vi "UI.vi"(0 "reference in":refnum<class "GUI Script Player.lvclass">, 5 "error in (no error)":errorcluster) -> (14 "reference out":refnum<class "GUI Script Player.lvclass">, 19 "error out":errorcluster)   [LabVIEW 2019, in "GUI Script Player.lvclass"]
uses:
  GUI Script Player.lvclass
  C:/Users/H4001/Documents/GitHub/H4000/src/GUI_class/GUI.lvclass
  GUI_class/GUI.lvclass/GUI.ctl
  ConfigJSON_class/ConfigJSON.lvclass
  TypeDef/Script.ctl
  TypeDef/Step.ctl
  TypeDef/Direction.ctl
  ConfigJSON_class/ConfigJSON.lvclass/ConfigJSON.ctl
  e526d8fc-7282-4644-9dda-8724ecf4fc0a.vi
  GUI_class/Set Win State.vi
  GUI_class/protected/GetSheredData.vi
  GUI_class/GUI.lvclass
panel:
  in  "Stop Button":bool
  in  "Start Button":bool
  out "String Indicator 2":string="Шаг 12/125"
  out "Horizontal Fill Indicator":dbl(slide)=29.646017699115045 scale=0.0..100.0
  out "XY Graph - Dark":cluster{"X":dbl[], "Y":dbl[]}[](graph) caption="Давление"
  out "Program name":string="Название"
  in  "Open":bool
  out "Steps":i32(listbox)
  # "Воспроизведение сценариев"
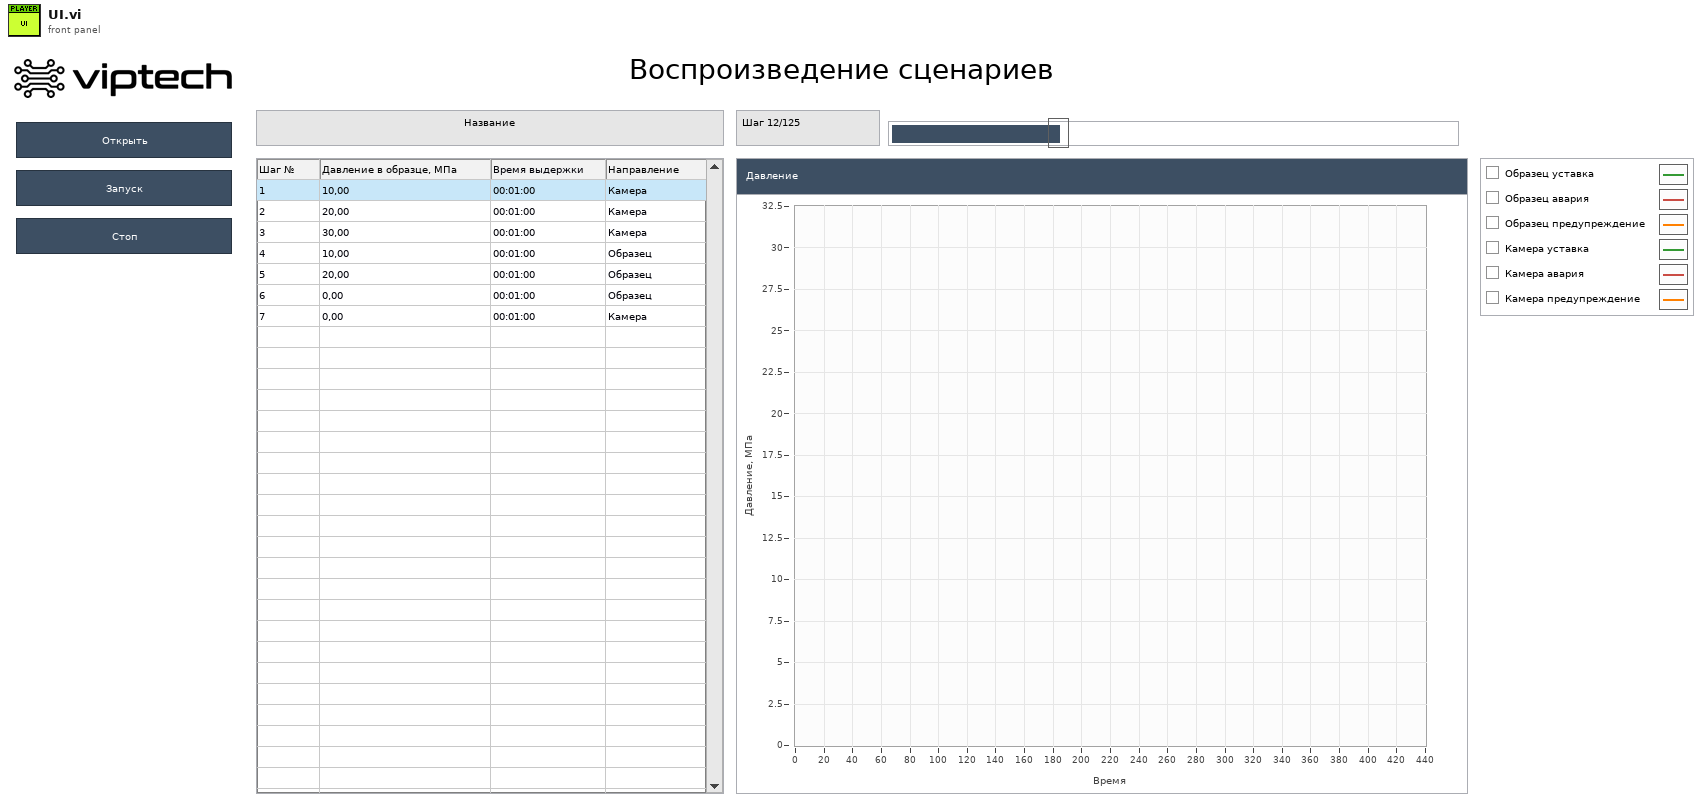
[diagram p1: front panel]
types:
  T1 = typedef "Script.ctl" = cluster{"Steps":T2[]}
  T2 = typedef "Step.ctl" = cluster{"Direction":T3, "Pressure MPa":dbl, "Time s":dbl, "Delta alarm MPa":dbl, "Delta warning MPa":dbl}
  T3 = typedef "Direction.ctl" = enum16{"None", "Chamber", "DUT"}
  T4 = enum32{"Invalid", "Standard", "Closed", "Hidden", "Minimized", "Maximized"}
  T5 = enum32{"invalid app kind", "Development System", "Run Time System", "Student Edition", "Embedded LabVIEW", "Evaluation", "Custom"}
  T6 = cluster{"Core":cluster{"Current VI Reference":refnum<vi>, "Close Panel on Exit?":bool}, "Dir Scripts":path, "Curr Script":T1, "selected path":path, "Steps ref":refnum<vi>}
  T7 = cluster{"Current VI Reference":refnum<vi>, "Close Panel on Exit?":bool}
  T8 = typedef "GUI Paths.ctl" = cluster{"Dir Data":path, "Dir Setting":path, "SensorLib":path, "Dir Scripts":path}
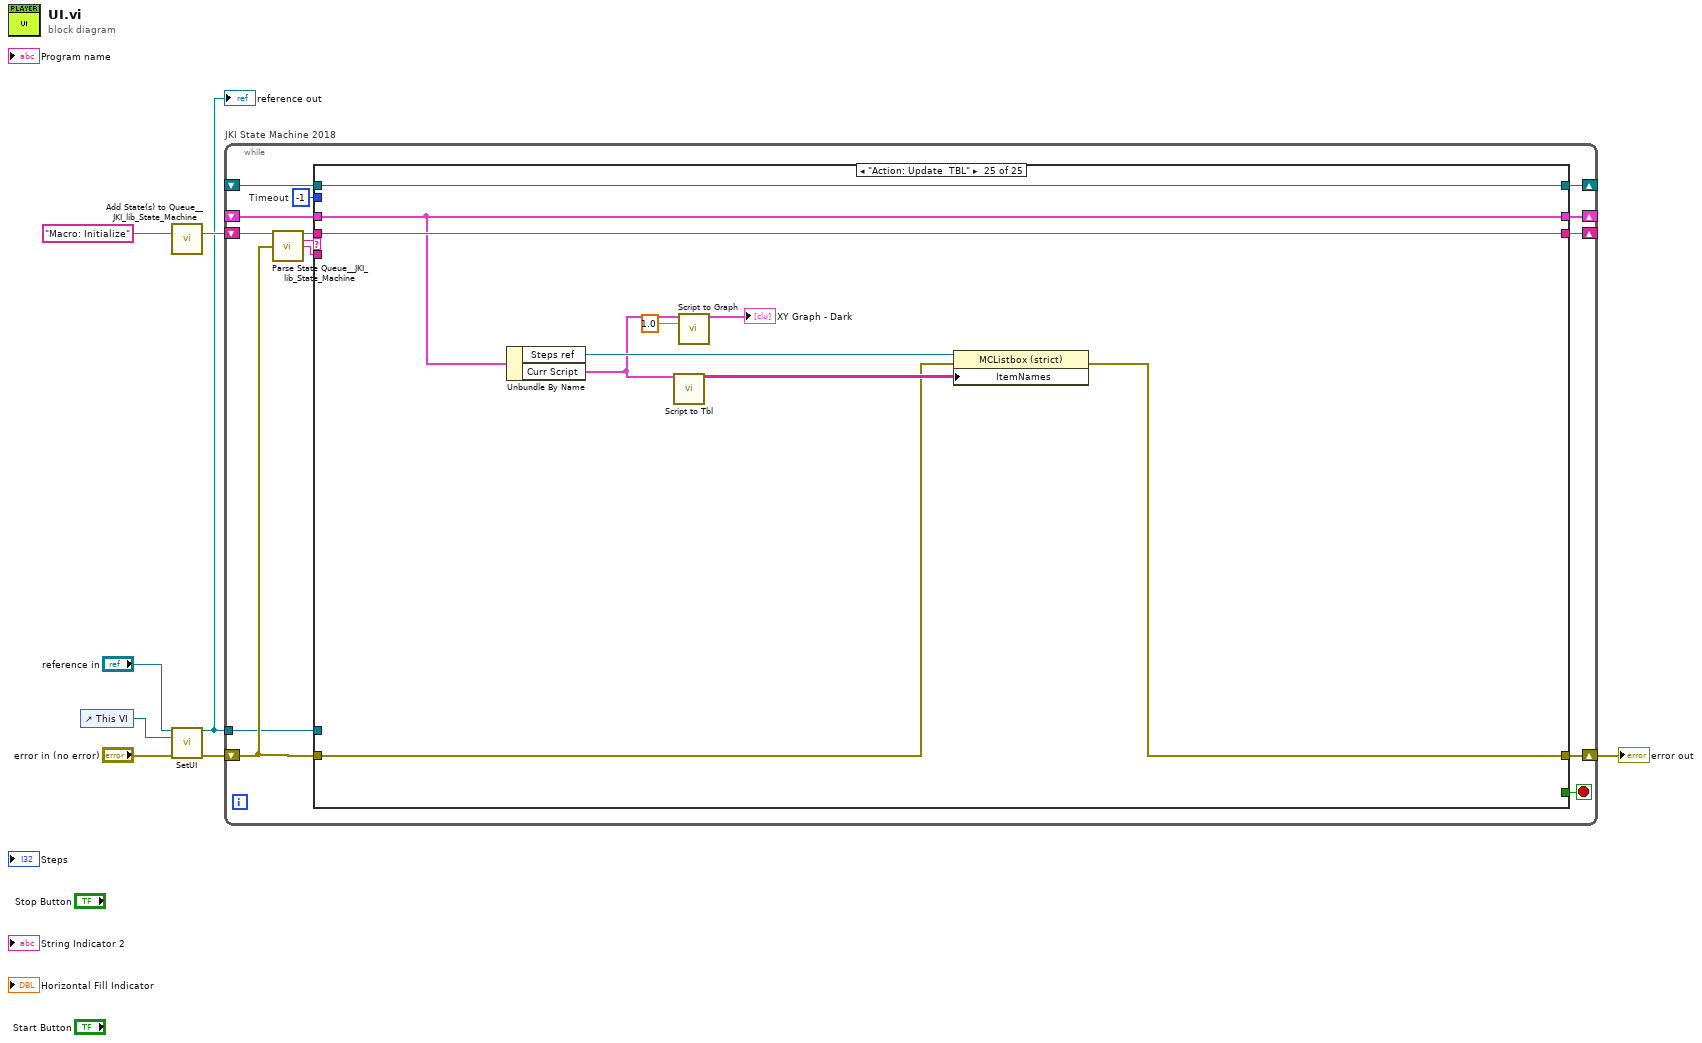
[diagram p0: block diagram]
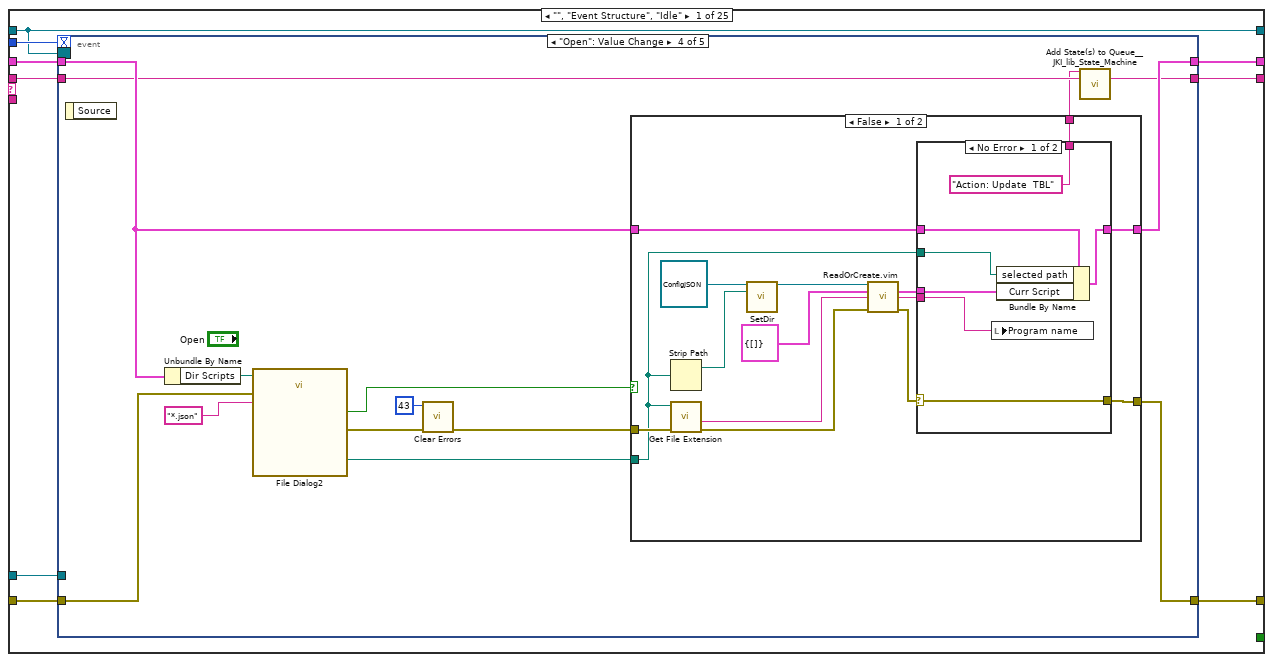
[diagram p2: hidden frame]
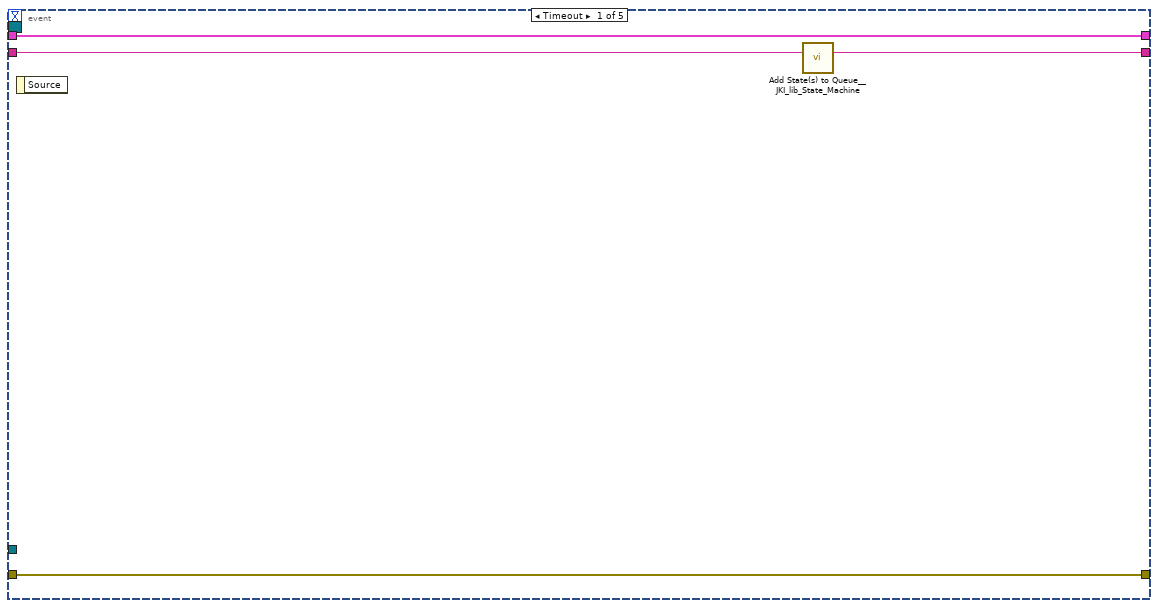
[diagram p3: hidden frame]
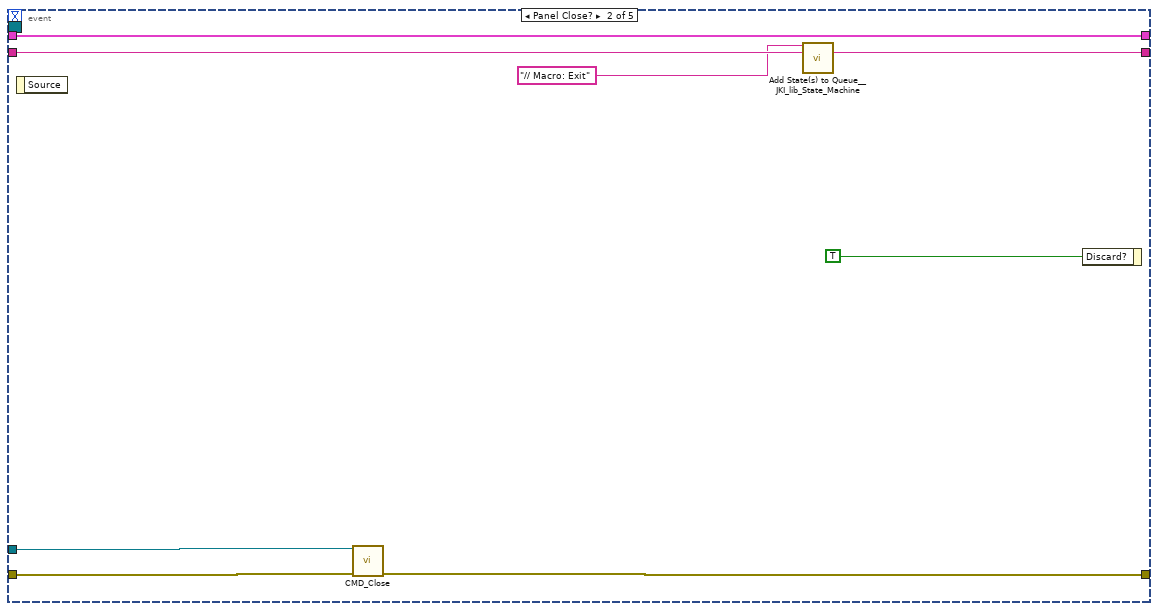
[diagram p4: hidden frame]
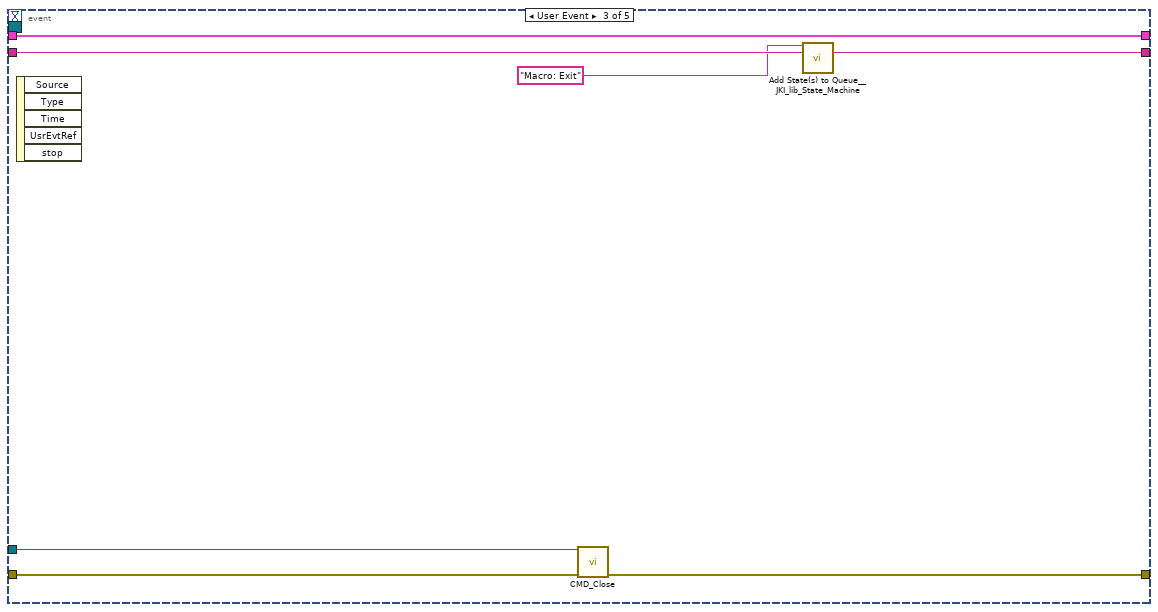
[diagram p5: hidden frame]
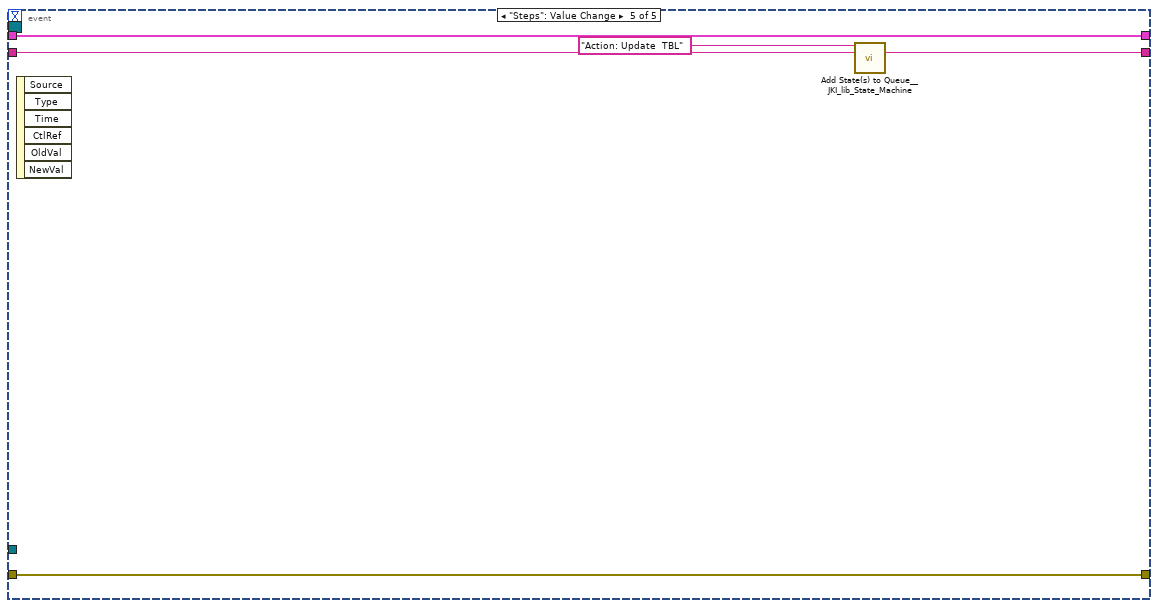
[diagram p8: hidden frame]
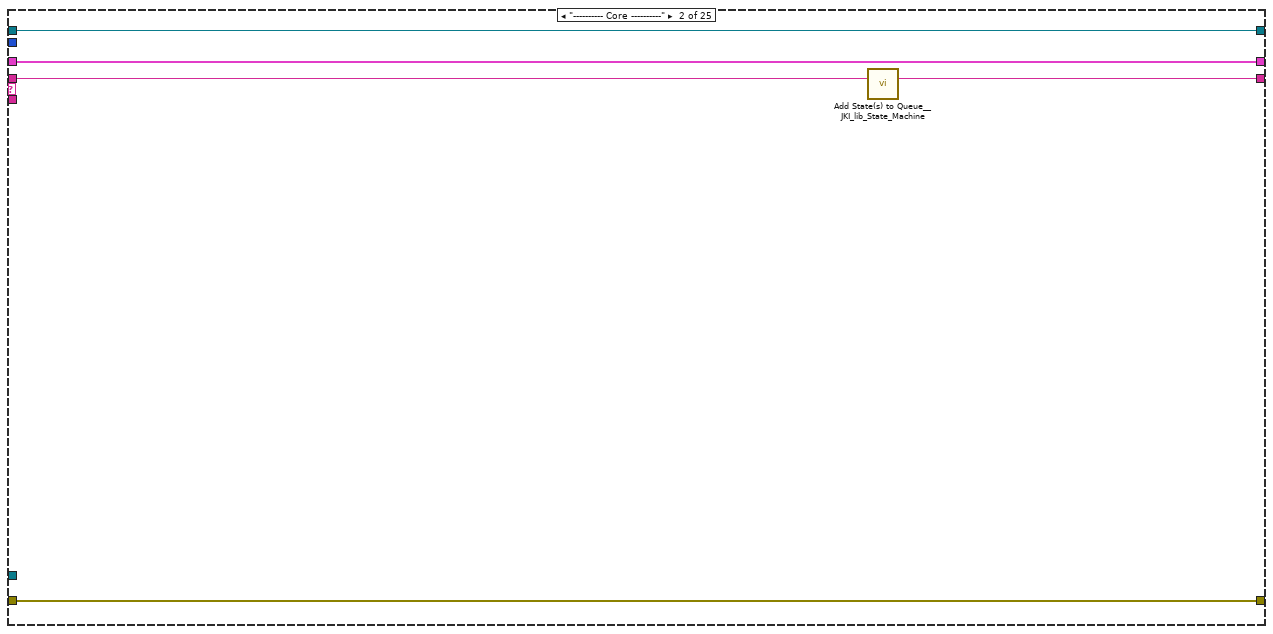
[diagram p9: hidden frame]
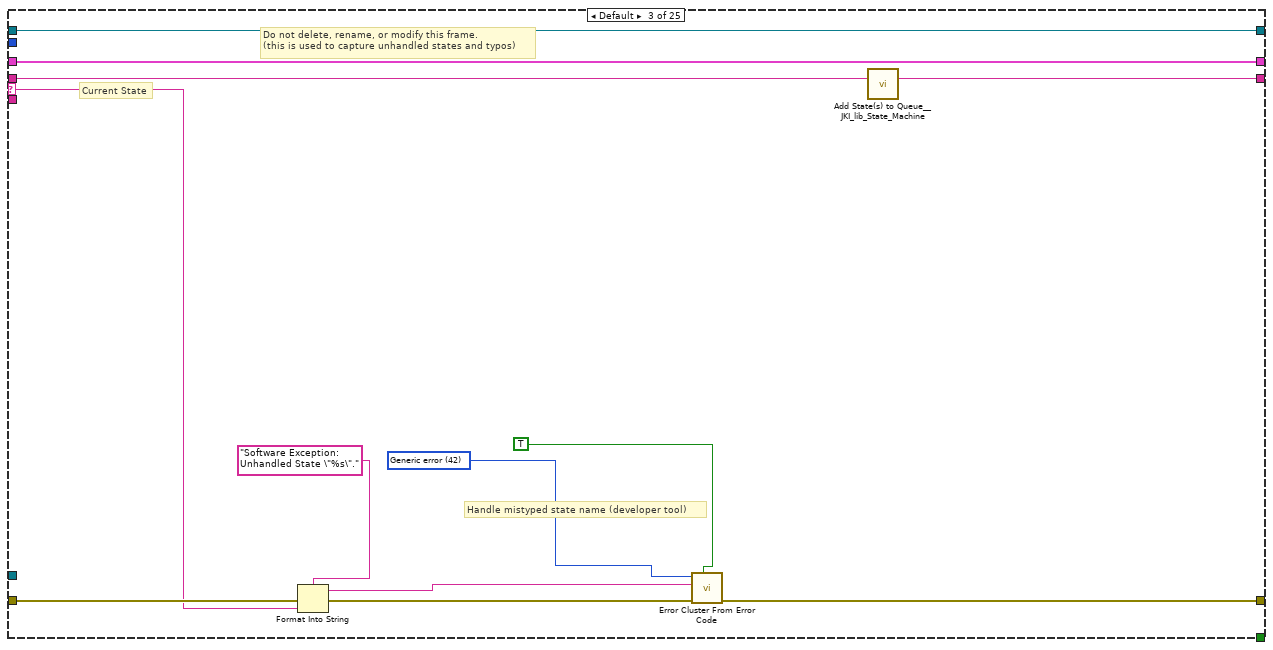
[diagram p10: hidden frame]
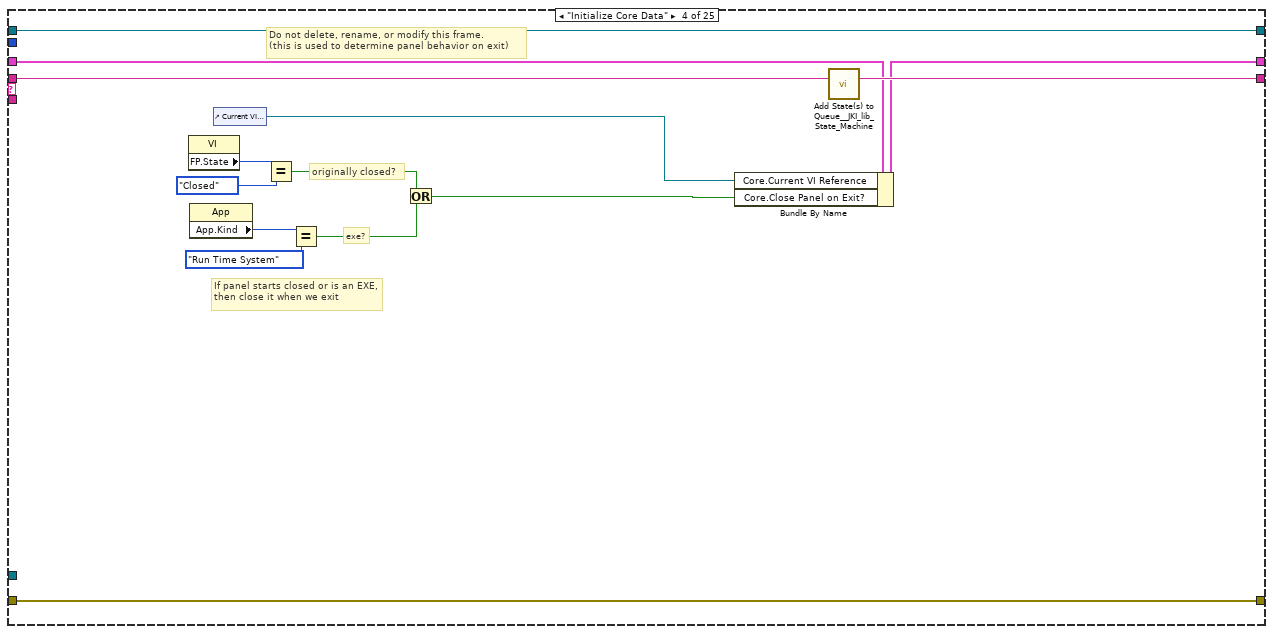
[diagram p11: hidden frame]
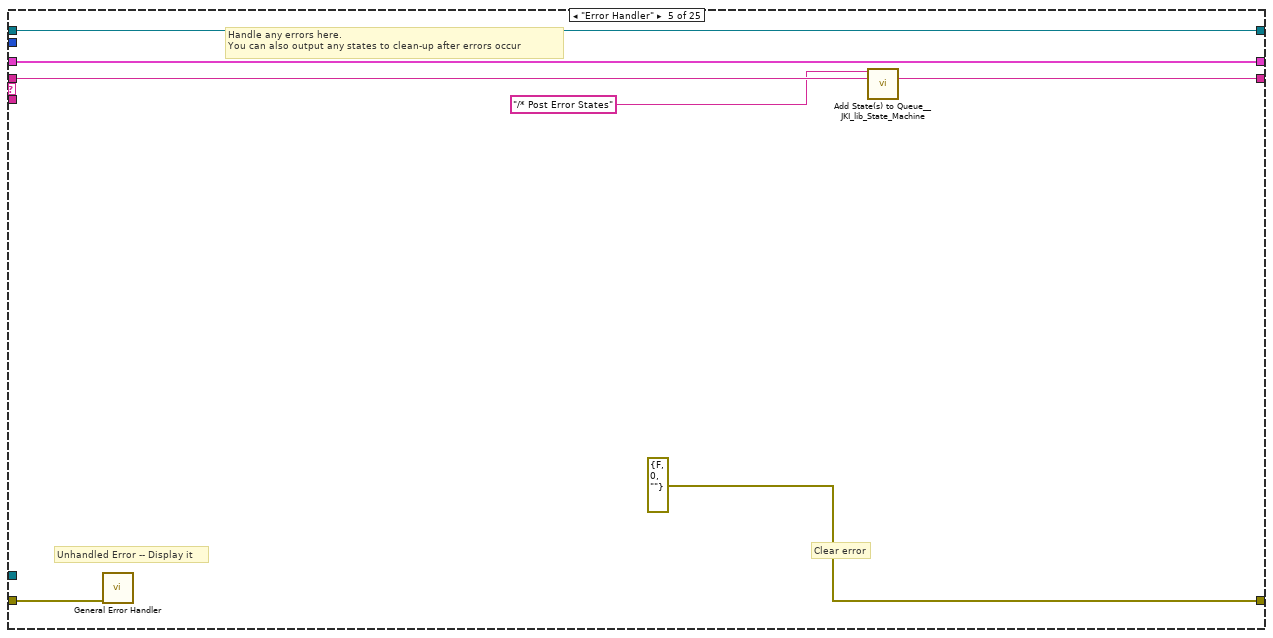
[diagram p12: hidden frame]
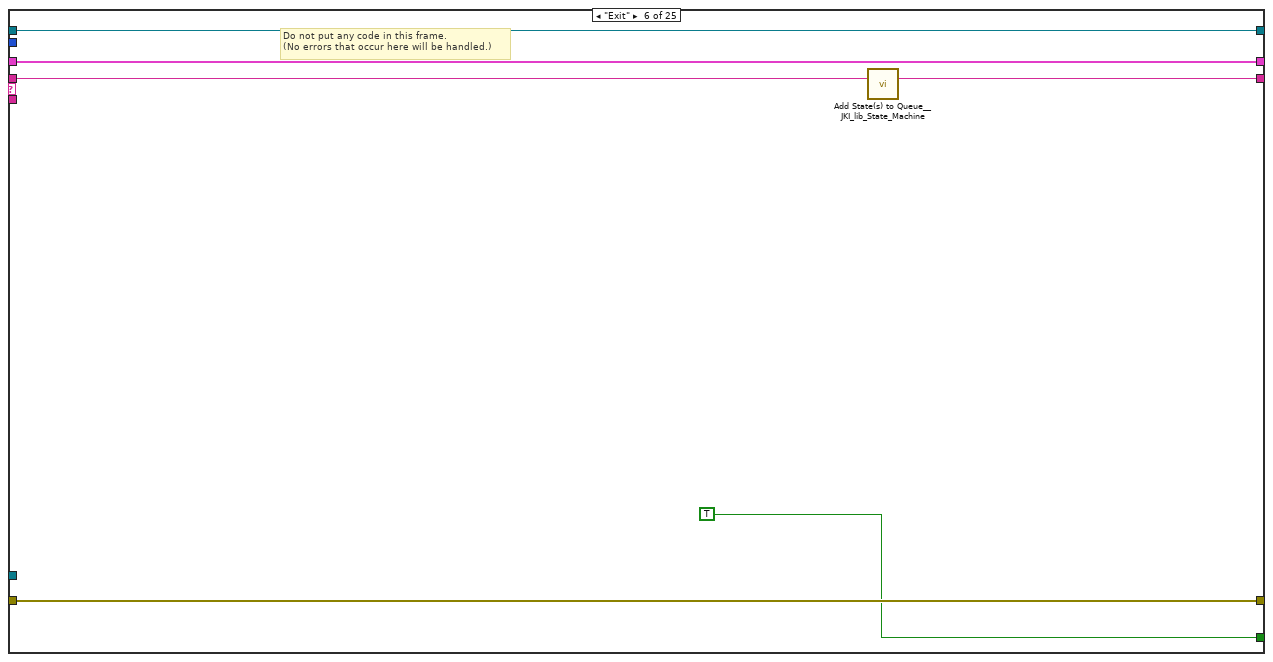
[diagram p13: hidden frame]
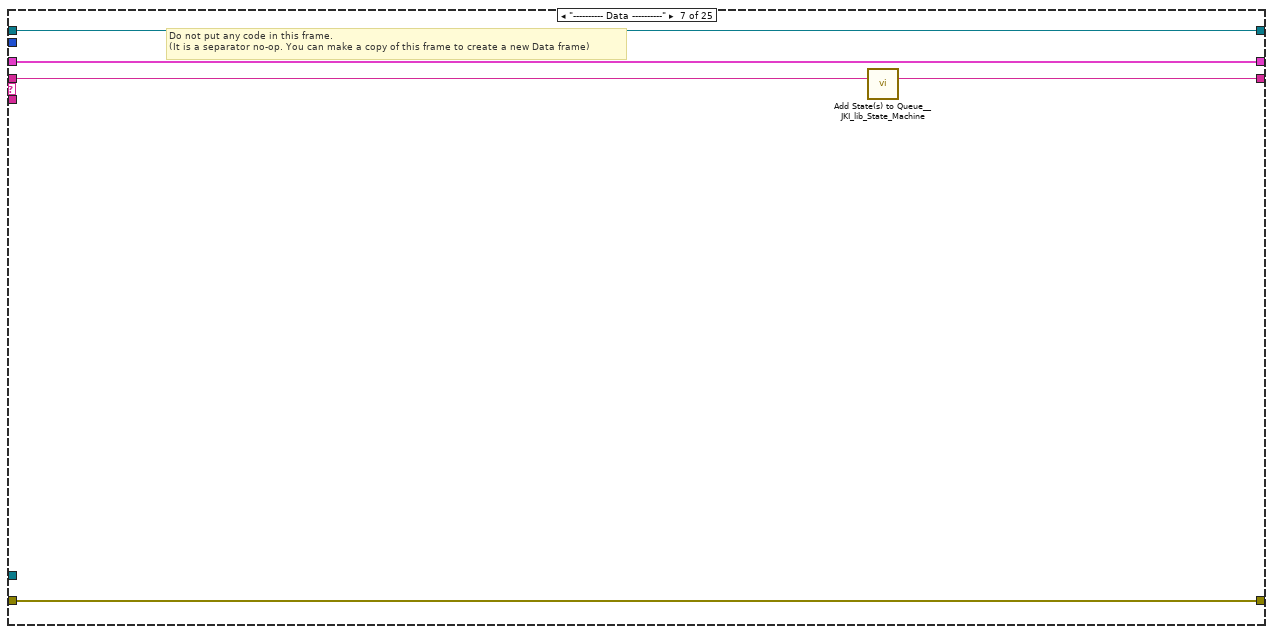
[diagram p14: hidden frame]
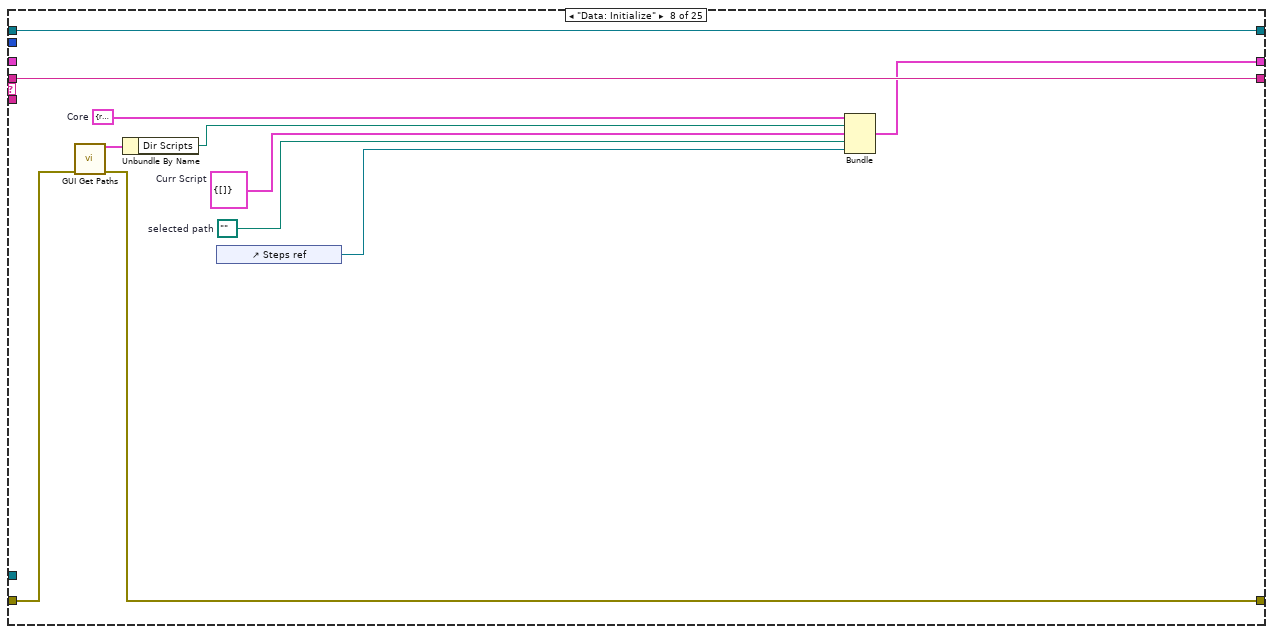
[diagram p15: hidden frame]
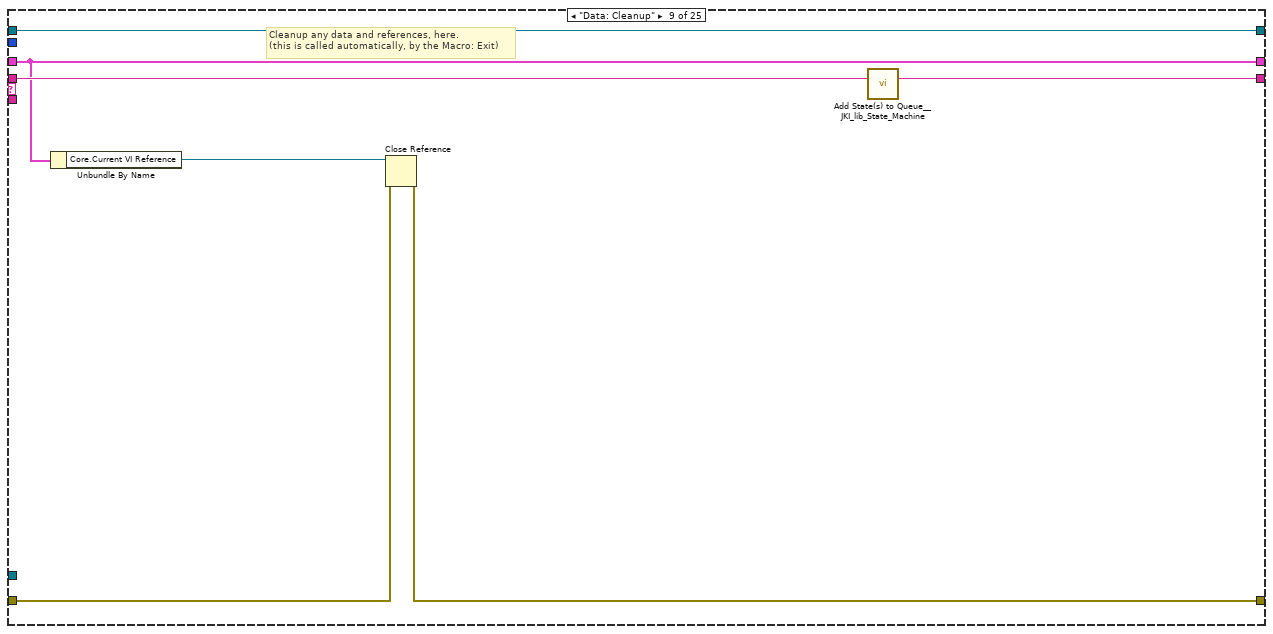
[diagram p16: hidden frame]
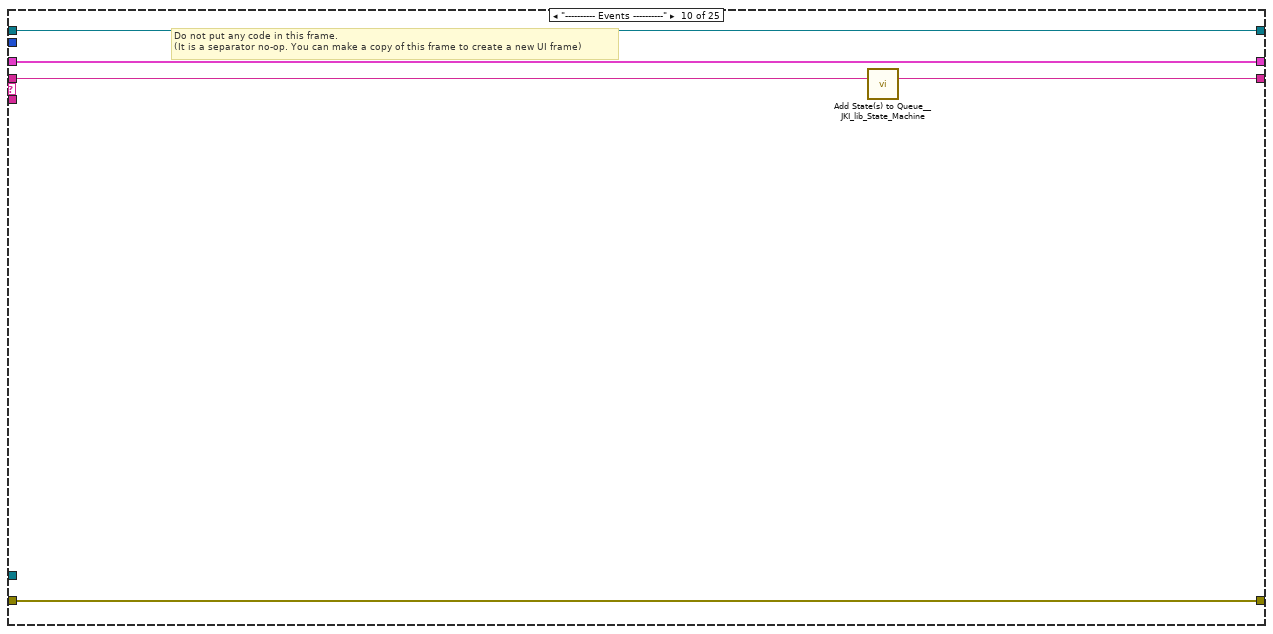
[diagram p17: hidden frame]
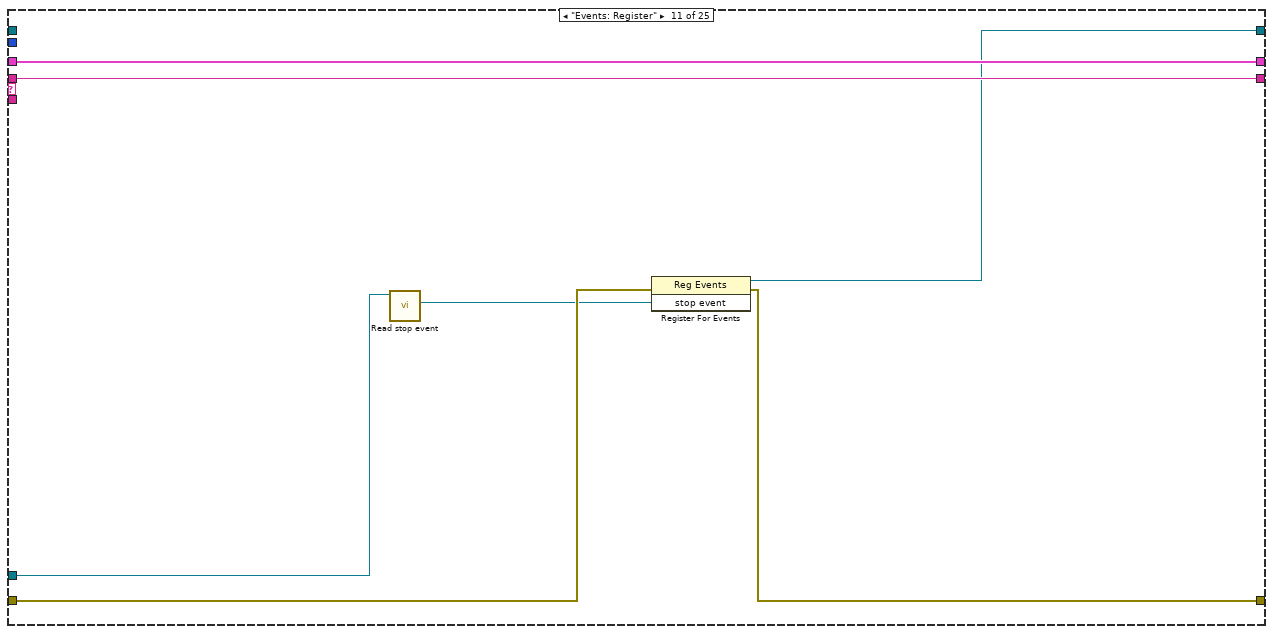
[diagram p18: hidden frame]
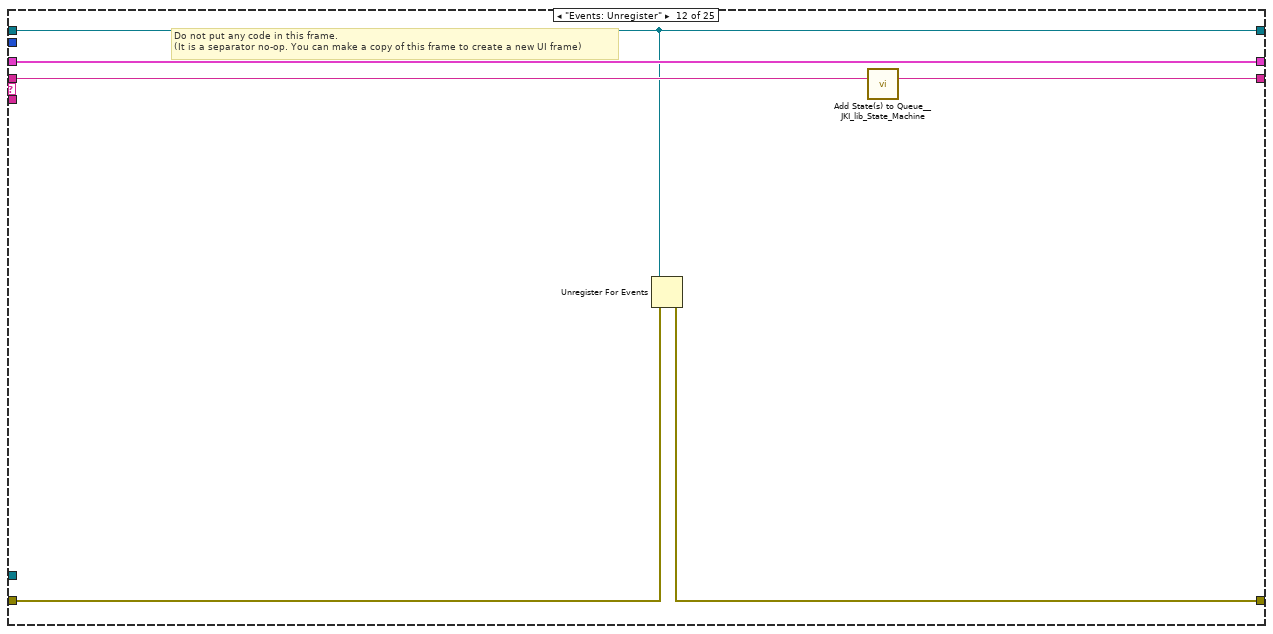
[diagram p19: hidden frame]
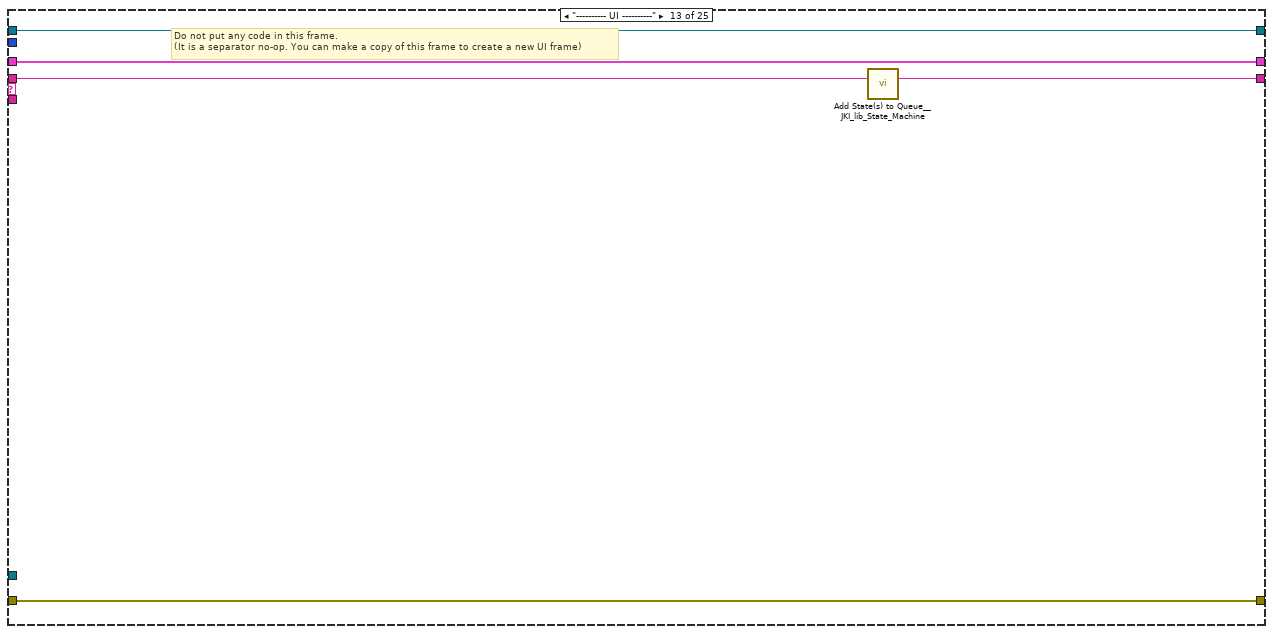
[diagram p20: hidden frame]
diagram:
  n1 = control-ref of="This VI"() -> (w3:refnum<vi>)
  n2 = call <vilib>:"Add State(s) to Queue__JKI_lib_State_Machine.vi"("State(s) in (\"\")"="Macro: Initialize") -> ("States Out"=w8:string)  [unwired: 14 in]
  n3 = call "SetUI.vi"("reference in"="reference in", "UI VI"=w3, "error in (no error)"="error in (no error)") -> ("reference out"=w1:refnum<class "GUI Script Player.lvclass">, "error out"=w2:errorcluster)  [unwired: 11 in]
  "reference out" <- w1
  n4 = while "JKI State Machine 2018" {
    shift-right: [w15] -> _
    shift-left: _ -> [w14]
    shift-right: [w18] -> w6
    shift-left: w2 -> [w12]
    shift-right: [w17] -> _
    shift-left: w8 -> [w19]
    tunnel: w1 -> [w11]
    shift-right: [w10] -> _
    shift-left: _ -> [w9]
    stop <- w16 stop-if-true
    w13 = -1  # Timeout
    n5 = call <vilib>:"Parse State Queue__JKI_lib_State_Machine.vi"("State Queue"=w19, "Error In (no error)"=w12) -> ("Remaining States"=w21:string, "Current State"=w22:string, "Arguments"=w20:string)  [unwired: 11 in]
    n6 = case shown="\"Action: Update  TBL\"" w22 {
      selector: w22 -> [_ _ w102 _ _ _ _ _ _ _ _ _ _ _ _ _ _ _ _ _ _ _ _ _ _]
      tunnel: w21 -> [w31 w100 w106 w126 w133 w139 w144 w155 w162 w167 w174 w180 w185 w189 w196 w208 w278 w284 w290 w302 w306 w311 w315 w320 w352]
      tunnel: w20 -> [_ _ _ _ _ _ _ _ _ _ _ _ _ _ w191 w202 _ _ _ _ _ _ _ _ _]
      tunnel: w14 -> [w29 w97 w104 w119 w130 w137 w141 _ w157 w164 w173 w178 w182 w188 w194 w204 w275 w281 w287 w299 w304 w309 w312 w317 w351]
      tunnel: [w28 w98 w108 w123 errorcluster {"status"=FALSE, "code"=0, "source"=""} ("error out") w136 w142 w148 w158 w165 w171 w175 w183 w187 w192 w205 w276 w282 w288 w300 w305 w308 w313 w318 w347] -> w18
      tunnel: w12 -> [w27 w98 w107 w123 w129 w136 w142 w150 w159 w165 w170 w176 w183 w187 w193 w206 w276 w282 w288 w300 w305 w307 w313 w318 w348]
      tunnel: [w30 w99 w105 w125 w132 w138 w143 w155 w161 w166 w174 w179 w184 w189 w195 w207 w277 w283 w289 w301 w306 w311 w315 w320 w352] -> w17
      tunnel: [_ _ _ _ _ TRUE _ _ _ _ _ _ _ _ _ _ _ _ _ _ _ _ _ _ _] -> w16
      tunnel: [w26 w97 w104 w124 w130 w137 w141 w154 w157 w164 w173 w178 w182 w188 w194 w204 w275 w281 w287 w299 w304 w309 w312 w317 w351] -> w15
      tunnel: w13 -> [w25 _ _ _ _ _ _ _ _ _ _ _ _ _ _ _ _ _ _ _ _ _ _ _ _]
      tunnel: w11 -> [w24 _ _ _ _ _ _ _ _ _ w169 _ _ _ _ _ _ _ _ _ _ _ _ _ _]
      tunnel: [w23 w96 w101 w113 w127 w134 w140 w152 w156 w163 w172 w177 w181 w186 w190 w201 w274 w279 w285 w292 w303 w310 w314 w319 w353] -> w10
      tunnel: w9 -> [w23 w96 w101 w113 w127 w134 w140 w152 w156 w163 _ w177 w181 w186 w190 w201 w274 w279 w285 w292 w303 w310 w314 w319 w353]
      frame "", "Event Structure", "Idle" {
        n7 = event shown="[3] \"Open\": Value Change" {
          selector: w23 -> [_ _ _ _ _]
          dyn-events: _ -> [_ _ _ _ _]
          timeout: w25 -> [_ _ _ _ _]
          tunnel: w31 -> [w35 w43 w50 w52 w92]
          tunnel: [w34 w42 w49 w53 w93] -> w30
          tunnel: w29 -> [w32 w41 w48 w55 w94]
          tunnel: [w33 w36 w44 w57 w95] -> w28
          tunnel: w27 -> [w33 w37 w45 w63 w95]
          tunnel: [w32 w41 w48 w54 w94] -> w26
          tunnel: w24 -> [_ w38 w46 _ _]
          event Timeout {
            n8 = event-data() -> ()  [unwired: 1 in, 1 out]
            n9 = call <vilib>:"Add State(s) to Queue__JKI_lib_State_Machine.vi"("State(s) in (\"\")"=w35) -> ("States Out"=w34:string)  [unwired: 14 in]
          }
          event Panel Close? {
            n10 = event-data() -> ()  [unwired: 1 in, 1 out]
            n11 = call "CMD_Close.vi"("reference in"=w38, "error in (no error)"=w37) -> ("error out"=w36:errorcluster)  [unwired: 12 in, 1 out]
            n12 = call <vilib>:"Add State(s) to Queue__JKI_lib_State_Machine.vi"("State(s) in Front (\"\")"="// Macro: Exit", "State(s) in (\"\")"=w43) -> ("States Out"=w42:string)  [unwired: 13 in]
            n13 = event-data("Discard?"=TRUE) -> ()  [unwired: 1 in, 1 out]
          }
          event User Event {
            n14 = event-data() -> ()  [unwired: 1 in, 5 out]
            n15 = call "CMD_Close.vi"("reference in"=w46, "error in (no error)"=w45) -> ("error out"=w44:errorcluster)  [unwired: 12 in, 1 out]
            n16 = call <vilib>:"Add State(s) to Queue__JKI_lib_State_Machine.vi"("State(s) in Front (\"\")"="Macro: Exit", "State(s) in (\"\")"=w50) -> ("States Out"=w49:string)  [unwired: 13 in]
          }
          event "Open": Value Change {
            n17 = event-data() -> ()  [unwired: 1 in, 1 out]
            n18 = Unbundle By Name(w55) -> ("Dir Scripts"=w64:path)
            n19 = call "File Dialog2"("start path"=w64, "error in"=w63, "pattern (all files)"="*.json") -> ("selected path"=w56:path, "cancelled"=w58:bool, "error out"=w60:errorcluster)  [unwired: 9 in, 1 out]
            n20 = call <vilib>:"Clear Errors.vi"("error in (no error)"=w60, "specific error code to clear (0: all)"=43) -> ("error out"=w59:errorcluster)  [unwired: 4 in, 1 out]
            n21 = case shown="False" w58 {
              tunnel: w59 -> [w76 w90]
              tunnel: [w71 w90] -> w57
              tunnel: w56 -> [w66 _]
              tunnel: w55 -> [w70 w89]
              tunnel: [w69 w89] -> w54
              tunnel: [w65 _] -> w51
              frame False {
                n22 = Strip Path(path=w66) -> (stripped path=w77:path)  [unwired: 1 out]
                n23 = call <vilib>:"Get File Extension.vi"("error in (no error)"=w76, "file"=w66) -> ("error out"=w73:errorcluster, "filename without extension"=w75:string)  [unwired: 5 in, 3 out]
                n24 = call "SetDir.vi"("reference in"=refnum<class "ConfigJSON.lvclass"> refnum ("ConfigJSON"), "Config Dir"=w77) -> ("JSON"=w78:refnum<class "ConfigJSON.lvclass">)  [unwired: 13 in]
                n25 = call "ReadOrCreate.vim"("reference in"=w78, "Type and Defaults"=T1 {"Steps"=[]} ("Script"), "Name"=w75, "error in (no error)"=w73) -> ("Data"=w68:T1, "Name dub"=w67:string, "error out"=w72:errorcluster)  [unwired: 7 in, 2 out]
                n26 = case shown="No Error" w72 {
                  selector: w72 -> [w83 w88]
                  tunnel: [w83 w88] -> w71
                  tunnel: w70 -> [w86 w87]
                  tunnel: [w85 w87] -> w69
                  tunnel: w68 -> [w84 _]
                  tunnel: w67 -> [w82 _]
                  tunnel: w66 -> [w81 _]
                  tunnel: ["Action: Update  TBL" ("State(s) in Front (\"\")") _] -> w65
                  frame No Error {
                    n27 = local write "Program name"(w82) -> ()
                    n28 = Bundle By Name(cluster=w86, "selected path"=w81, "Curr Script"=w84) -> (w85:T6)
                  }
                  frame Error {
                  }
                }
              }
              frame True {
              }
            }
            n29 = call <vilib>:"Add State(s) to Queue__JKI_lib_State_Machine.vi"("State(s) in Front (\"\")"=w51, "State(s) in (\"\")"=w52) -> ("States Out"=w53:string)  [unwired: 13 in]
          }
          event "Steps": Value Change {
            n30 = event-data() -> ()  [unwired: 1 in, 6 out]
            n31 = call <vilib>:"Add State(s) to Queue__JKI_lib_State_Machine.vi"("State(s) in Front (\"\")"="Action: Update  TBL" ("State(s) in Front (\"\")"), "State(s) in (\"\")"=w92) -> ("States Out"=w93:string)  [unwired: 13 in]
          }
        }
      }
      frame "---------- Core ----------" {
        n32 = call <vilib>:"Add State(s) to Queue__JKI_lib_State_Machine.vi"("State(s) in (\"\")"=w100) -> ("States Out"=w99:string)  [unwired: 14 in]
      }
      frame Default {
        w111 = 42 items=["No error", "Argument error", "Memory is full", "Out of zone", "End of file", "File already open", "Generic file I/O error", "File not found", "File permission error", "Disk is full", "Duplicate path", "Too many files open", "System feature not enabled", "Resource file not found", "Cannot add resource", "Resource not found", "Image not found", "Image memory error", "Pen does not exist", "Config type invalid", "Config token not found", "Config parse error", "Config memory error", "Bad external code format", "Bad external code offset", "External code not present", "Null window", "Destroy window error", "Null menu", "Print aborted", "Bad print record", "Print driver error", "Windows error during printing", "Memory error during printing", "Print dialog error", "Generic print error", "Invalid device refnum", "Device not found", "Device parameter error", "Device unit error", "Cannot open device", "Device call aborted", "Generic error", "Cancelled by user", "Object ID too low", "Object ID too high", "Object not in heap", "Unknown heap", "Unknown object (invalid DefProc)", "Unknown object (DefProc not in table)", "Message out of range", "Invalid (null) method", "Unknown message", "Manager call not supported", "Bad address", "Network operation in progress", "Network operation timed out", "Connection is busy", "Network attribute not supported", "Network error", "Address in use", "System out of memory", "Connection aborted", "Connection refused", "Not connected", "Already connected", "Connection closed", "Initialization error (interapplication manager)", "Bad occurrence", "Wait on unbound occurrence handler", "Occurrence queue overflow", "Datalog type conflict", "Unused", "Unrecognized type (interapplication manager)", "Memory corrupt", "Failed to make temporary DLL", "Old CIN version", "Drag socket not found", "Failed to load drop-object", "Failed to register OLE object", "Failed to release OLE object", "Format specifier type mismatch", "Unknown format specifier", "Too few format specifiers", "Too many format specifiers", "Scan failed", "Newer CIN version", "Error converting to variant", "Runtime menu error", "Password tampered", "Variant attribute not found", "Incompatible variant data type", "Event data is not available", "Event Store is not present", "Occurrence is not found", "Event Queue is not created", "Event info is not available", "Refnum passed is NULL", "Error retrieving Class GUID", "Error retrieving CoClass GUID", "Error retrieving TypeLib GUID.", "Bad built application magic bytes.", "Specific driver is different from the specific driver associated with the Logical Name.", "There is no session opened to the class driver.", "Max Error", "MAX - Error with config objects", "MAX - Error loading configuration", "MAX - Group not supported"]
        # "Current State"
        # "Do not delete, rename, or modify this frame.\n(this is used to capture unhandled states and typos)"
        # "Handle mistyped state name (developer tool)"
        n33 = Format Into String(format string="Software Exception: Unhandled State \"%s\"." ("message"), error in=w107, w102) -> (resulting string=w110:string, error out=w109:errorcluster)  [unwired: 1 in]
        n34 = call <vilib>:"Error Cluster From Error Code.vi"("show call chain? (False)"=TRUE, "error in (no error)"=w109, "error message (\"\")"=w110, "error code (0)"=w111) -> ("error out"=w108:errorcluster)  [unwired: 5 in]
        n35 = call <vilib>:"Add State(s) to Queue__JKI_lib_State_Machine.vi"("State(s) in (\"\")"=w106) -> ("States Out"=w105:string)  [unwired: 14 in]
      }
      frame "Initialize Core Data" {
        # "Do not delete, rename, or modify this frame.\n(this is used to determine panel behavior on exit)"
        # "originally closed?"
        # "exe?"
        # "If panel starts closed or is an EXE, then close it when we exit"
        n36 = property class="VI"() -> ("FP.State"=w116:T4)  [unwired: 2 in, 2 out]
        n37 = property class="App"() -> ("App.Kind"=w122:T5)  [unwired: 2 in, 2 out]
        n38 = control-ref of="Current VI Reference"() -> (w117:refnum<vi>)
        n39 = Equal?(x=w116, y=T4."Closed" ("Front Panel Window:State")) -> (x = y?=w114:bool)
        n40 = Equal?(x=w122, y=T5."Run Time System" ("Application:Kind")) -> (x = y?=w120:bool)
        n41 = Or(x=w114, y=w120) -> (x .or. y?=w118:bool)
        n42 = Bundle By Name(cluster=w119, "Core.Current VI Reference"=w117, "Core.Close Panel on Exit?"=w118) -> (w124:T6)
        n43 = call <vilib>:"Add State(s) to Queue__JKI_lib_State_Machine.vi"("State(s) in (\"\")"=w126) -> ("States Out"=w125:string)  [unwired: 14 in]
      }
      frame "Error Handler" {
        # "Unhandled Error -- Display it"
        # "Handle any errors here.\nYou can also output any states to clean-up after errors occur"
        # "Clear error"
        n44 = call <vilib>:"General Error Handler.vi"("error in (no error)"=w129) -> ()  [unwired: 10 in, 5 out]
        n45 = call <vilib>:"Add State(s) to Queue__JKI_lib_State_Machine.vi"("State(s) in Front (\"\")"="/* Post Error States", "State(s) in (\"\")"=w133) -> ("States Out"=w132:string)  [unwired: 13 in]
      }
      frame "Exit" {
        # "Do not put any code in this frame.\n(No errors that occur here will be handled.)"
        n46 = call <vilib>:"Add State(s) to Queue__JKI_lib_State_Machine.vi"("State(s) in (\"\")"=w139) -> ("States Out"=w138:string)  [unwired: 14 in]
      }
      frame "---------- Data ----------" {
        # "Do not put any code in this frame.\n(It is a separator no-op. You can make a copy of this frame to create a new Data frame)"
        n47 = call <vilib>:"Add State(s) to Queue__JKI_lib_State_Machine.vi"("State(s) in (\"\")"=w144) -> ("States Out"=w143:string)  [unwired: 14 in]
      }
      frame "Data: Initialize" {
        w146 = path ""  # selected path
        w147 = T1 {"Steps"=[]}  # Curr Script
        w153 = T7 {"Current VI Reference"=refnum, "Close Panel on Exit?"=FALSE}  # Core
        n48 = call "GUI Get Paths.vi"("error in (no error)"=w150) -> ("Paths"=w151:T8, "error out"=w148:errorcluster)  [unwired: 13 in]
        n49 = Unbundle By Name(w151) -> ("Dir Scripts"=w149:path)
        n50 = control-ref of="Steps ref"() -> (w145:refnum<vi>)
        n51 = Bundle("Core"=w153, "Dir Scripts"=w149, "Curr Script"=w147, "selected path"=w146, "Steps ref"=w145) -> (w154:T6)  [unwired: 1 in]
      }
      frame "Data: Cleanup" {
        # "Cleanup any data and references, here.\n(this is called automatically, by the Macro: Exit)"
        n52 = Unbundle By Name(w157) -> ("Core.Current VI Reference"=w160:refnum<vi>)
        n53 = Close Reference(reference=w160, error in (no error)=w159) -> (error out=w158:errorcluster)
        n54 = call <vilib>:"Add State(s) to Queue__JKI_lib_State_Machine.vi"("State(s) in (\"\")"=w162) -> ("States Out"=w161:string)  [unwired: 14 in]
      }
      frame "---------- Events ----------" {
        # "Do not put any code in this frame.\n(It is a separator no-op. You can make a copy of this frame to create a new UI frame)"
        n55 = call <vilib>:"Add State(s) to Queue__JKI_lib_State_Machine.vi"("State(s) in (\"\")"=w167) -> ("States Out"=w166:string)  [unwired: 14 in]
      }
      frame "Events: Register" {
        n56 = call "Read stop event.vi"("GUI in"=w169) -> ("stop event"=w168:refnum<user-event>)  [unwired: 8 in, 2 out]
        n57 = register-events(error in=w170, w168) -> (reference out=w172:refnum<event-registration>, error out=w171:errorcluster)  [unwired: 1 in]
      }
      frame "Events: Unregister" {
        # "Do not put any code in this frame.\n(It is a separator no-op. You can make a copy of this frame to create a new UI frame)"
        n58 = Unregister For Events(event registration refnum=w177, error in=w176) -> (error out=w175:errorcluster)
        n59 = call <vilib>:"Add State(s) to Queue__JKI_lib_State_Machine.vi"("State(s) in (\"\")"=w180) -> ("States Out"=w179:string)  [unwired: 14 in]
      }
      frame "---------- UI ----------" {
        # "Do not put any code in this frame.\n(It is a separator no-op. You can make a copy of this frame to create a new UI frame)"
        n60 = call <vilib>:"Add State(s) to Queue__JKI_lib_State_Machine.vi"("State(s) in (\"\")"=w185) -> ("States Out"=w184:string)  [unwired: 14 in]
      }
      frame "UI: Initialize" {
      }
      frame "UI: Cursor Set" {
        # "Argument"
        # "Set and Unset Cursor Busy.\n(Usage: \"UI: Cursor Set >> Busy|Idle\")"
        n61 = case shown="\"Idle\", Default" w191 {
          tunnel: w193 -> [w198 w200]
          tunnel: [w197 w199] -> w192
          frame "Idle", Default {
            n62 = call <vilib>:"Unset Busy.vi"("error in (no error)"=w198) -> ("error out"=w197:errorcluster)  [unwired: 10 in]
          }
          frame "Busy" {
            n63 = call <vilib>:"Set Busy.vi"("error in (no error)"=w200) -> ("error out"=w199:errorcluster)  [unwired: 9 in, 1 out]
          }
        }
        n64 = call <vilib>:"Add State(s) to Queue__JKI_lib_State_Machine.vi"("State(s) in (\"\")"=w196) -> ("States Out"=w195:string)  [unwired: 14 in]
      }
      frame "UI: Front Panel State" {
        # "Argument"
        # "Set Front Panel Open or Closed\n(Usage: \"UI: Front Panel State >> Open|Close\")"
        n65 = Unbundle By Name(w204) -> ("Core.Current VI Reference"=w203:refnum<vi>)
        n66 = case shown="\"Minimize\", \"Minimized\"" w202 {
          tunnel: w206 -> [w214 w229 w240 w253 w266]
          tunnel: [w216 w230 w242 w255 w268] -> w205
          tunnel: w203 -> [w215 w227 w241 w254 w267]
          frame "Open", "Standard", Default {
            w209 = T4."Standard" ("State")
            n67 = property class="VI"(reference=w215, error in=w214) -> (reference out=w212:refnum<vi>, error out=w213:errorcluster, "FP.State"=w211:T4)
            n68 = Not Equal?(x=w211, y=w209) -> (x != y?=w210:bool)
            n69 = case shown="True" w210 {
              tunnel: [w220 w222] -> w216
              tunnel: w213 -> [w219 w222]
              tunnel: w212 -> [w218 _]
              tunnel: w209 -> [w217 _]
              frame True {
                n70 = invoke class="VI" method="FP.Open"(reference=w218, error in=w219, "Activate"=TRUE, "State"=w217) -> (error out=w220:errorcluster)  [unwired: 1 in, 4 out]
              }
              frame False {
              }
            }
          }
          frame "Close", "Closed" {
            n71 = property class="VI"(reference=w227, error in=w229) -> (reference out=w226:refnum<vi>, error out=w228:errorcluster, "FP.State"=w224:T4)
            n72 = Not Equal?(x=w224, y=T4."Closed" ("Front Panel Window:State")) -> (x != y?=w223:bool)
            n73 = case shown="True" w223 {
              tunnel: [w231 w234] -> w230
              tunnel: w228 -> [w231 w233]
              tunnel: w226 -> [_ w232]
              frame False {
              }
              frame True {
                n74 = invoke class="VI" method="FP.Close"(reference=w232, error in=w233) -> (error out=w234:errorcluster)  [unwired: 1 in, 2 out]
              }
            }
          }
          frame "Hidden", "Hide" {
            w235 = T4."Hidden" ("State")
            n75 = property class="VI"(reference=w241, error in=w240) -> (reference out=w238:refnum<vi>, error out=w239:errorcluster, "FP.State"=w237:T4)
            n76 = Not Equal?(x=w237, y=w235) -> (x != y?=w236:bool)
            n77 = case shown="True" w236 {
              tunnel: [w246 w247] -> w242
              tunnel: w239 -> [w245 w247]
              tunnel: w238 -> [w244 _]
              tunnel: w235 -> [w243 _]
              frame True {
                n78 = invoke class="VI" method="FP.Open"(reference=w244, error in=w245, "State"=w243) -> (error out=w246:errorcluster)  [unwired: 2 in, 4 out]
              }
              frame False {
              }
            }
          }
          frame "Minimize", "Minimized" {
            w248 = T4."Minimized" ("State")
            n79 = property class="VI"(reference=w254, error in=w253) -> (reference out=w251:refnum<vi>, error out=w252:errorcluster, "FP.State"=w250:T4)
            n80 = Not Equal?(x=w250, y=w248) -> (x != y?=w249:bool)
            n81 = case shown="True" w249 {
              tunnel: [w259 w260] -> w255
              tunnel: w252 -> [w258 w260]
              tunnel: w251 -> [w257 _]
              tunnel: w248 -> [w256 _]
              frame True {
                n82 = invoke class="VI" method="FP.Open"(reference=w257, error in=w258, "State"=w256) -> (error out=w259:errorcluster)  [unwired: 2 in, 4 out]
              }
              frame False {
              }
            }
          }
          frame "Maximize", "Maximized" {
            w261 = T4."Maximized" ("State")
            n83 = property class="VI"(reference=w267, error in=w266) -> (reference out=w264:refnum<vi>, error out=w265:errorcluster, "FP.State"=w263:T4)
            n84 = Not Equal?(x=w263, y=w261) -> (x != y?=w262:bool)
            n85 = case shown="True" w262 {
              tunnel: [w272 w273] -> w268
              tunnel: w265 -> [w271 w273]
              tunnel: w264 -> [w270 _]
              tunnel: w261 -> [w269 _]
              frame True {
                n86 = invoke class="VI" method="FP.Open"(reference=w270, error in=w271, "State"=w269) -> (error out=w272:errorcluster)  [unwired: 2 in, 4 out]
              }
              frame False {
              }
            }
          }
        }
        n87 = call <vilib>:"Add State(s) to Queue__JKI_lib_State_Machine.vi"("State(s) in (\"\")"=w208) -> ("States Out"=w207:string)  [unwired: 14 in]
      }
      frame "---------- Macro ----------" {
        # "Do not put any code in this frame.\n(It is a separator no-op. You can make a copy of this frame to create a new Macro frame)"
        n88 = call <vilib>:"Add State(s) to Queue__JKI_lib_State_Machine.vi"("State(s) in (\"\")"=w278) -> ("States Out"=w277:string)  [unwired: 14 in]
      }
      frame "Macro: Initialize" {
        n89 = call <vilib>:"Add State(s) to Queue__JKI_lib_State_Machine.vi"("State(s) in Front (\"\")"="Data: Initialize\nInitialize Core Data\nEvents: Register\nUI: Initialize\n// UI: Front Panel State >> Open\n\n\nAction: Read Config\nAction: Update Indicators\nAction: Update  TBL", "State(s) in (\"\")"=w284) -> ("States Out"=w283:string)  [unwired: 13 in]
      }
      frame "Macro: Update" {
        n90 = call <vilib>:"Add State(s) to Queue__JKI_lib_State_Machine.vi"("State(s) in Front (\"\")"="Action: Update Indicators\n", "State(s) in (\"\")"=w290) -> ("States Out"=w289:string)  [unwired: 13 in]
      }
      frame "Macro: Exit" {
        # "Exit Macro\n(This is called once, when the VI exits)"
        n91 = Unbundle By Name(w299) -> ("Core.Close Panel on Exit?"=w298:bool)
        n92 = Select(t="UI: Front Panel State >> Close", s=w298, f="") -> (s? t:f=w295:string)
        n93 = call <vilib>:"Add State(s) to Queue__JKI_lib_State_Machine.vi"("State(s) in Front (\"\")"="Action: Write Config", "State(s) in (\"\")"=w295, "State(s) at Back (\"\")"="Data: Cleanup\nEvents: Unregister\nExit") -> ("States Out"=w293:string)  [unwired: 12 in]
        n94 = call <vilib>:"Add State(s) to Queue__JKI_lib_State_Machine.vi"("State(s) in Front (\"\")"=w293, "State(s) in (\"\")"=w302) -> ("States Out"=w301:string)  [unwired: 13 in]
      }
      frame "---------- Action ----------" {
      }
      frame "Action: Read Config" {
        n95 = Merge Errors(w307) -> (w308:errorcluster)
      }
      frame "Action: Write Config" {
      }
      frame "Action: Update Indicators" {
        n96 = Unbundle By Name(w317) -> ("Curr Script.Steps"=w316:T2[])
        n97 = disable-structure shown="Disabled" {
          disable-tunnel: w316 -> [w321 _]
          frame Disabled {
            n98 = for {
              tunnel: w321 -> [w341] mode=indexing
              i -> [w324]
              n99 = Unbundle By Name(w341) -> ("Pressure MPa"=w340:dbl, "Direction"=w337:T3, "Time s"=w335:dbl)
              n100 = Increment(x=w324) -> (x+1=w323:i32)
              n101 = case shown="\"DUT\"" w337 {
                tunnel: ["Образец" "Камера"] -> w336
                frame "DUT" {
                }
                frame "Chamber" {
                }
              }
              n102 = Quotient & Remainder(x=w335, y=60.0) -> (x-y*floor(x/y)=w330:dbl, floor(x/y)=w332:dbl)
              n103 = Number To Fractional String(number=w340, precision (6)=i16 2) -> (F-format string=w338:string)  [unwired: 2 in]
              n104 = Number To Fractional String(number=w323, precision (6)=i16 0) -> (F-format string=w322:string)  [unwired: 2 in]
              n105 = Number To Fractional String(number=w332, precision (6)=i16 0) -> (F-format string=w329:string)  [unwired: 2 in]
              n106 = Number To Fractional String(number=w330, precision (6)=i16 0) -> (F-format string=w328:string)  [unwired: 2 in]
              n107 = Concatenate Strings(w329, ":" ("string"), w328) -> (w326:string)
              n108 = Build Array(w322, w338, w336, w326) -> ()  [unwired: 1 out]
            }
          }
          frame Enabled {
          }
        }
      }
      frame "Action: Update  TBL" {
        n109 = Unbundle By Name(w351) -> ("Steps ref"=w350:refnum<vi>, "Curr Script"=w346:T1)
        n110 = call "Script to Tbl.vi"("Script"=w346) -> ("Tbl"=w349:string[][])  [unwired: 14 in]
        n111 = call "Script to Graph.vi"("Script"=w346, "tr"=1.0) -> ("XY Data"=→"XY Graph - Dark":cluster{"X":dbl[], "Y":dbl[]}[])  [unwired: 13 in]
        n112 = property class="MCListbox (strict)"(reference=w350, error in=w348, "ItemNames"=w349) -> (error out=w347:errorcluster)  [unwired: 1 out]
      }
    }
  }
  "error out" <- w6
